vi "Pre Launch Init.vi"(11 "Data Logger Actor in":refnum<class "Data Logger Actor.lvclass">) -> (0 "error out":errorcluster, 3 "Data Logger Actor out":refnum<class "Data Logger Actor.lvclass">)   [LabVIEW 2024, in "Data Logger Actor.lvlib" / "Data Logger Actor.lvclass"]
doc: "Initializes the panel actor. Creates the Panel Helper.\n\n----\nPlease see the following web address for additional documentation and tutorial information:\nhttp://www.mooregoodideas.com/mgi-panel-manager/\n\nAuthor: Derek Trepanier\n\nCopyright (c) 2018, Moore Good Ideas, Inc.\n\nAll rights reserved.\n\nRedistribution and use in source and binary forms, with or without modification, are permitted provided that the following conditions are met:\n\n * Redistributions of source code must retain the above copyright notice, this list of conditions and the following disclaimer.\n * Redistributions in binary form must reproduce the above copyright notice, this list of conditions and the following disclaimer in the documentation and/or other materials provided with the distribution.\n * Neither the name of Moore Good Ideas, Inc. nor the names of its contributors may be used to endorse or promote products derived from this software without specific prior written permission.\n\nTHIS SOFTWARE IS PROVIDED BY THE COPYRIGHT HOLDERS AND CONTRIBUTORS \"AS IS\" AND ANY EXPRESS OR IMPLIED WARRANTIES, INCLUDING, BUT NOT LIMITED TO, THE IMPLIED WARRANTIES OF MERCHANTABILITY AND FITNESS FOR A PARTICULAR PURPOSE ARE DISCLAIMED. IN NO EVENT SHALL THE COPYRIGHT OWNER OR CONTRIBUTORS BE LIABLE FOR ANY DIRECT, INDIRECT, INCIDENTAL, SPECIAL, EXEMPLARY, OR CONSEQUENTIAL DAMAGES (INCLUDING, BUT NOT LIMITED TO, PROCUREMENT OF SUBSTITUTE GOODS OR SERVICES; LOSS OF USE, DATA, OR PROFITS; OR BUSINESS INTERRUPTION) HOWEVER CAUSED AND ON ANY THEORY OF LIABILITY, WHETHER IN CONTRACT, STRICT LIABILITY, OR TORT (INCLUDING NEGLIGENCE OR OTHERWISE) ARISING IN ANY WAY OUT OF THE USE OF THIS SOFTWARE, EVEN IF ADVISED OF THE POSSIBILITY OF SUCH DAMAGE."
uses:
  Data Logger Actor.lvclass
  Data Logger Actor.lvclass/Data Logger Actor.ctl
  <vilib>/MGI/Panel Manager/Panel Actor/Panel Actor/Panel Actor.lvclass
  Data Sink/IData Sink/IData Sink.lvclass
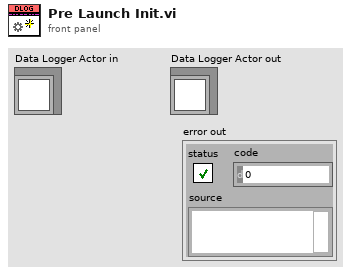
[diagram p1: front panel]
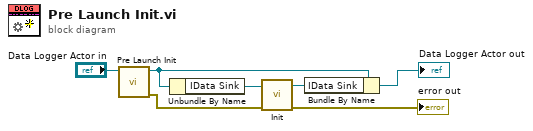
[diagram p0: block diagram]
diagram:
  n1 = call-parent "Pre Launch Init.vi"("Panel Actor in"="Data Logger Actor in") -> ("error out"=w4:errorcluster, "Panel Actor out"=w2:refnum<class "Data Logger Actor.lvclass">)  [unwired: 9 in]
  n2 = Unbundle By Name(w2) -> ("IData Sink"=w7:refnum<class "IData Sink.lvclass">)
  n3 = call-dynamic "Init.vi"("error in"=w4, "IData Sink in"=w7) -> ("error out"=→"error out":errorcluster, "IData Sink out"=w6:refnum<class "IData Sink.lvclass">)  [unwired: 8 in]
  n4 = Bundle By Name(cluster=w2, "IData Sink"=w6) -> (→"Data Logger Actor out":refnum<class "Data Logger Actor.lvclass">)
